vi "JKI Temelate.vi"() -> ()   [LabVIEW 2021]
uses:
  <userlib>/sushu/sushu.lvlib
panel:
  out "error out":errorcluster
  in  "error in (no error)":errorcluster
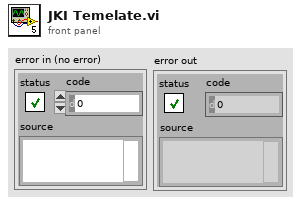
[diagram p1: front panel]
types:
  T1 = cluster{"Core":cluster{"Current VI Reference":refnum<vi>, "Close Panel on Exit?":bool}, "VI Name":string}
  T2 = enum32{"Invalid", "Standard", "Closed", "Hidden", "Minimized", "Maximized"}
  T3 = enum32{"invalid app kind", "Development System", "Run Time System", "Student Edition", "Embedded LabVIEW", "Evaluation", "Custom"}
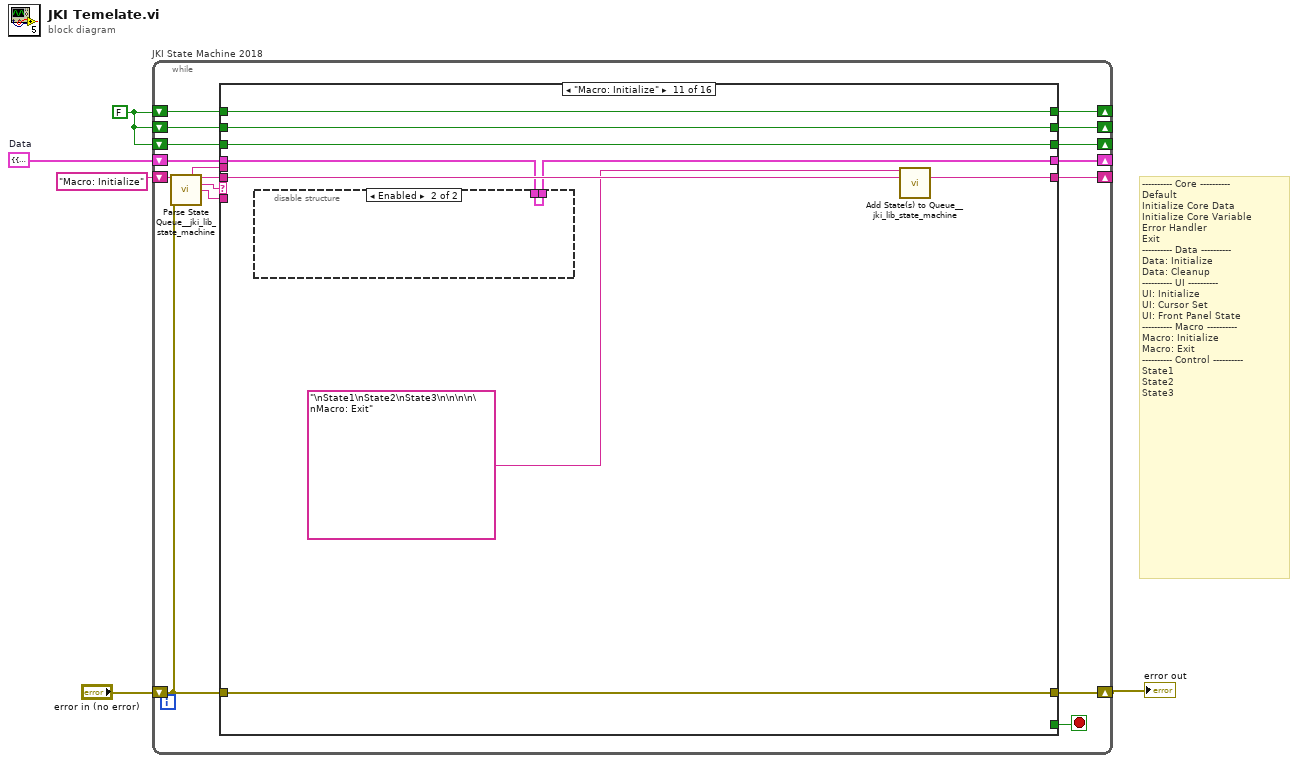
[diagram p0: block diagram]
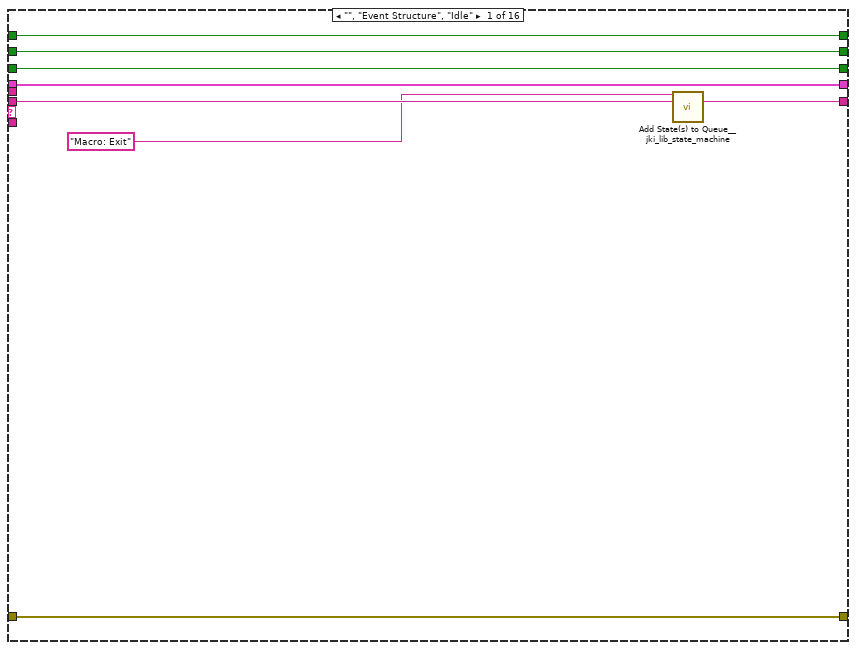
[diagram p2: hidden frame]
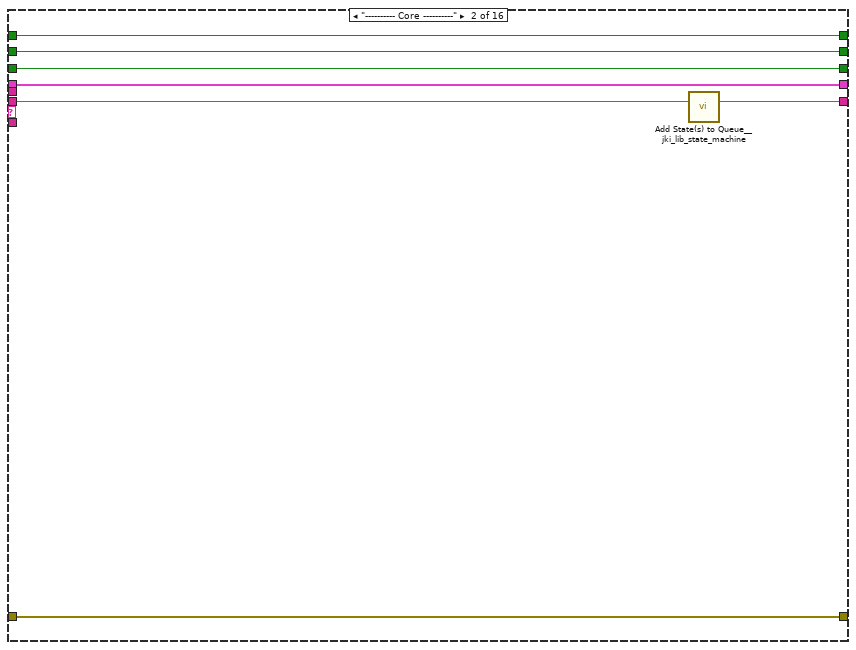
[diagram p3: hidden frame]
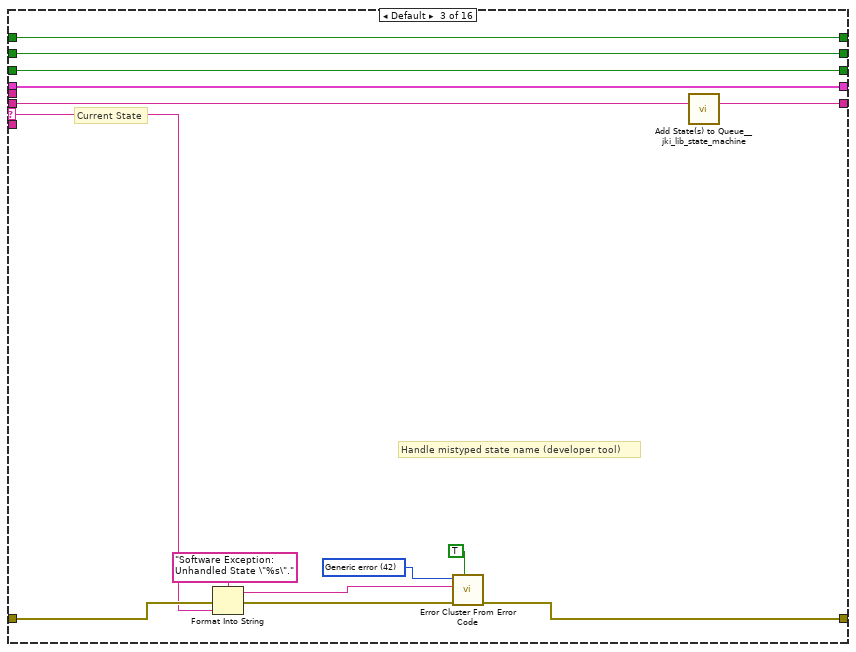
[diagram p4: hidden frame]
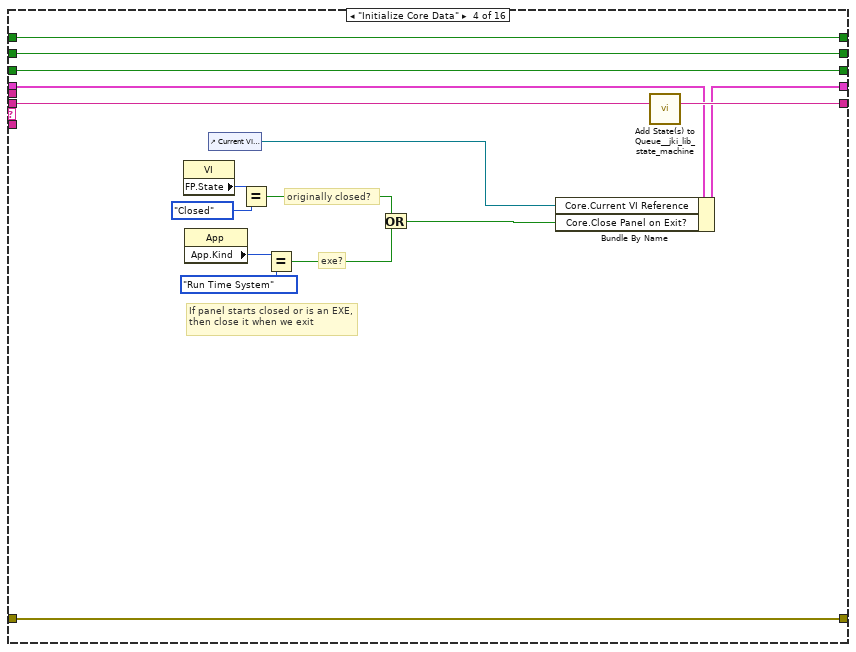
[diagram p5: hidden frame]
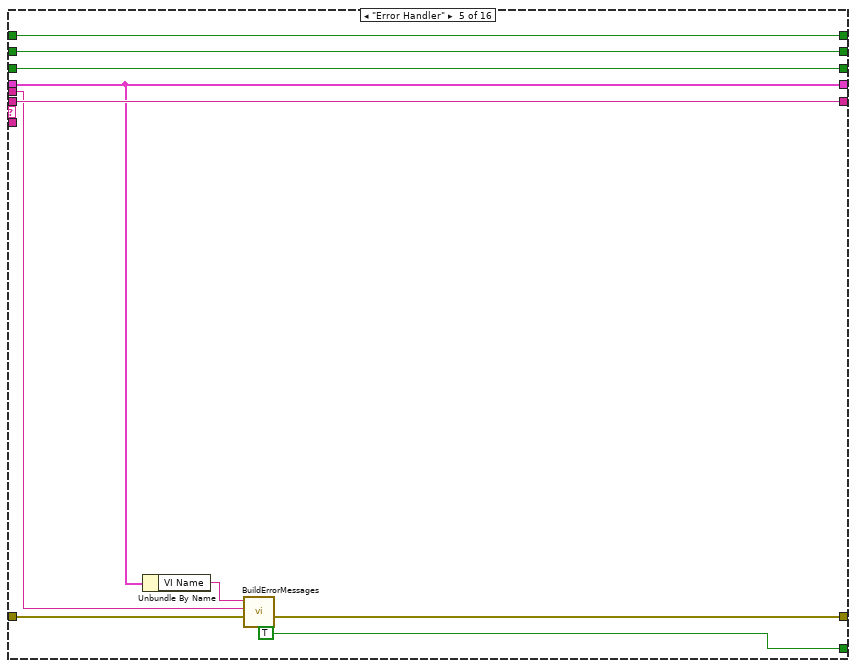
[diagram p6: hidden frame]
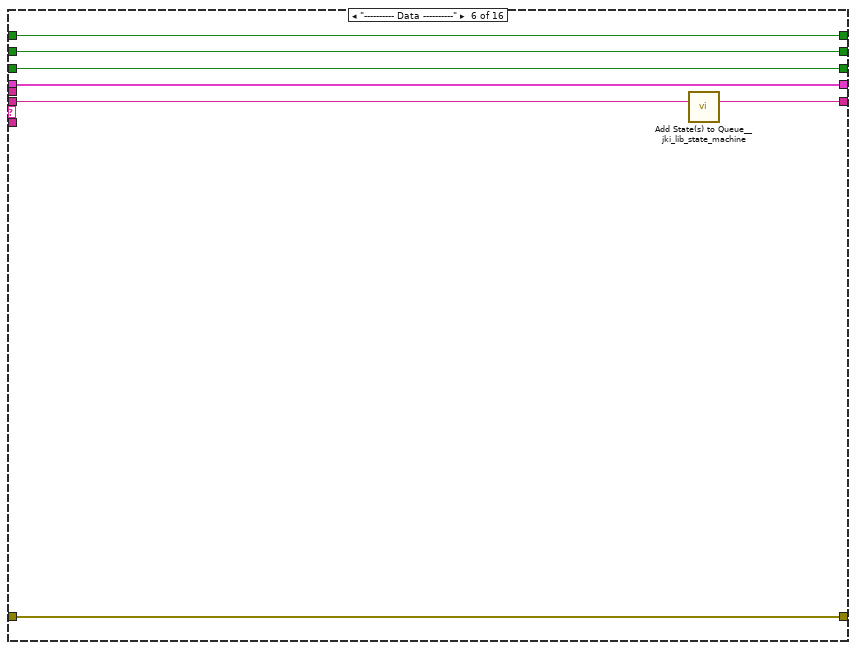
[diagram p7: hidden frame]
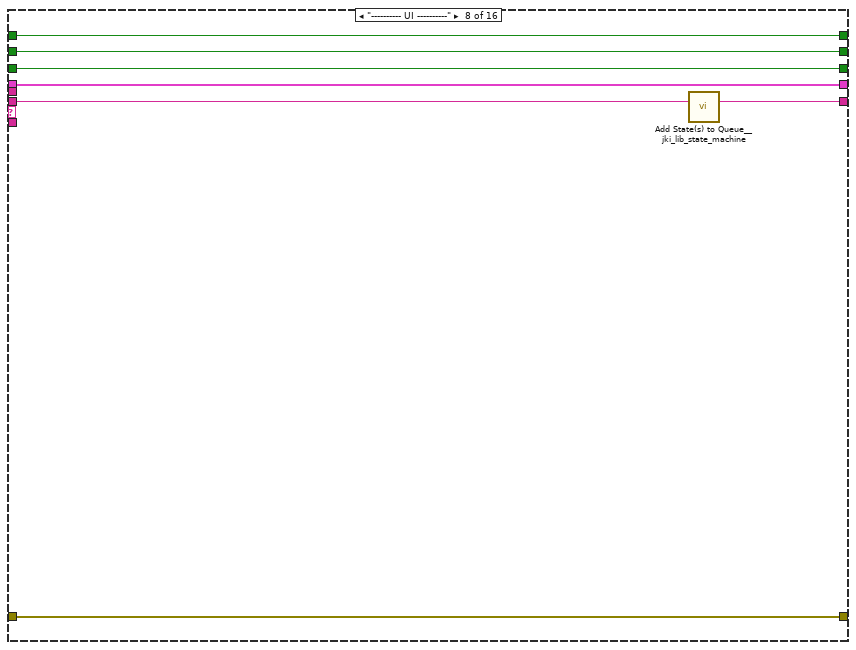
[diagram p9: hidden frame]
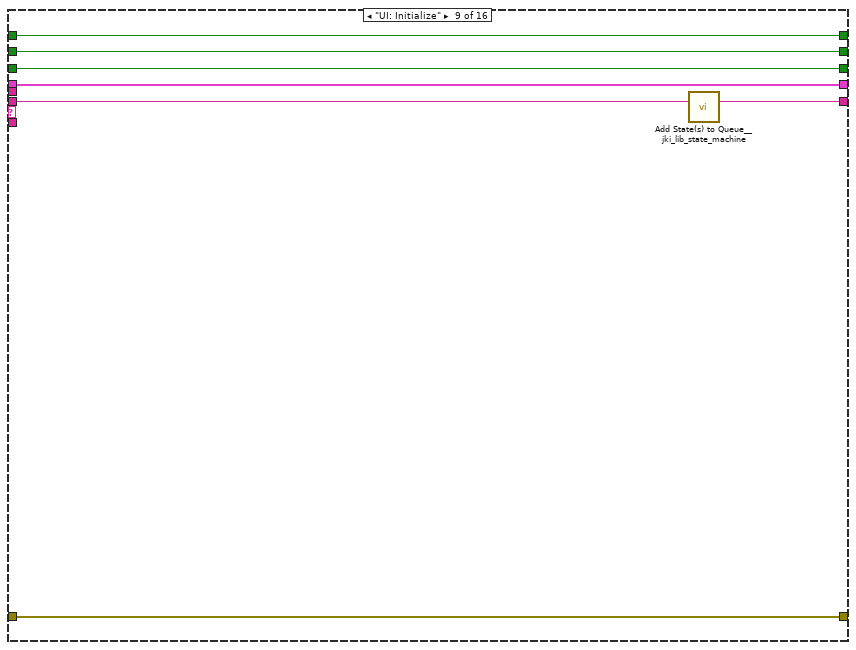
[diagram p10: hidden frame]
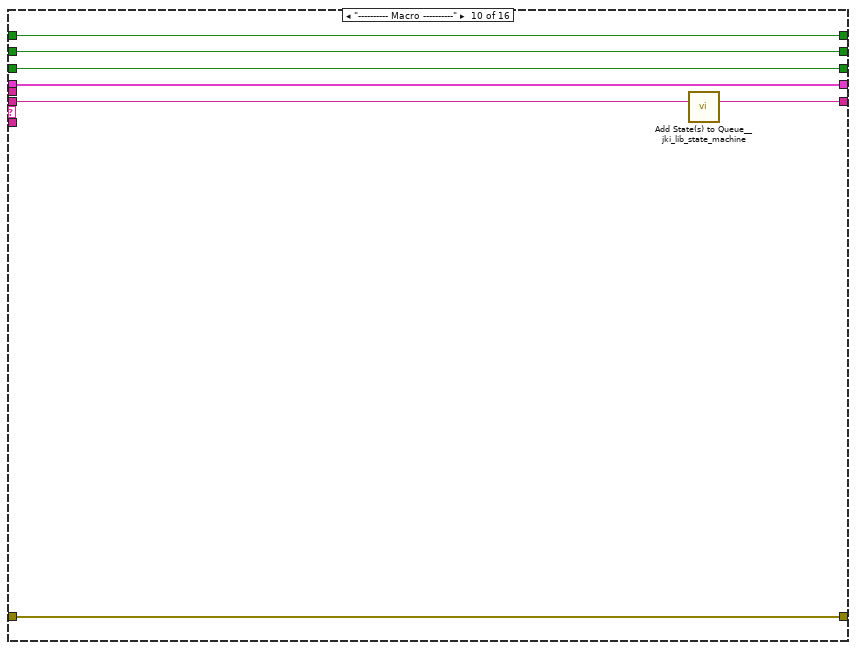
[diagram p11: hidden frame]
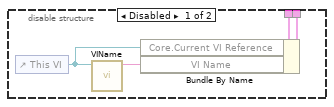
[diagram p12: hidden frame]
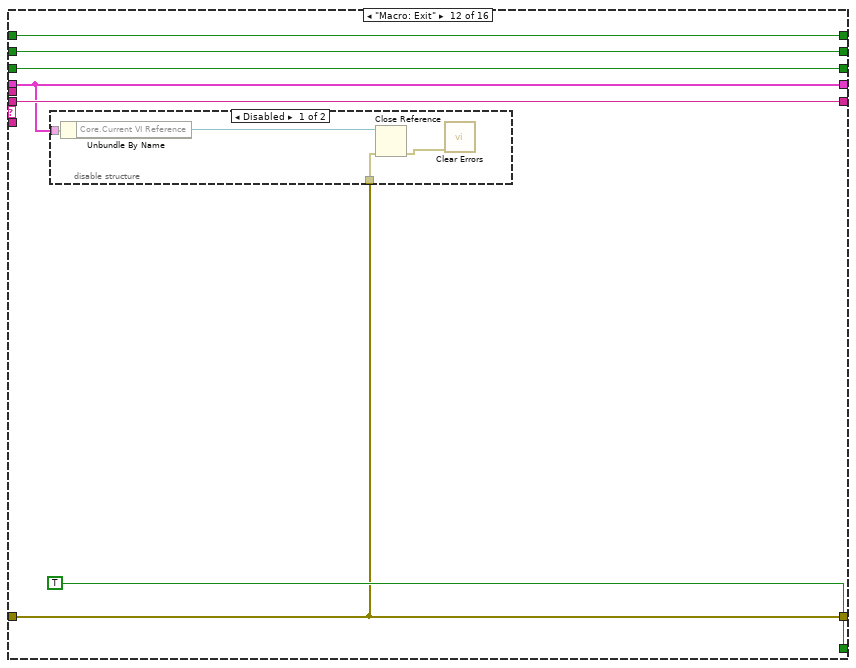
[diagram p13: hidden frame]
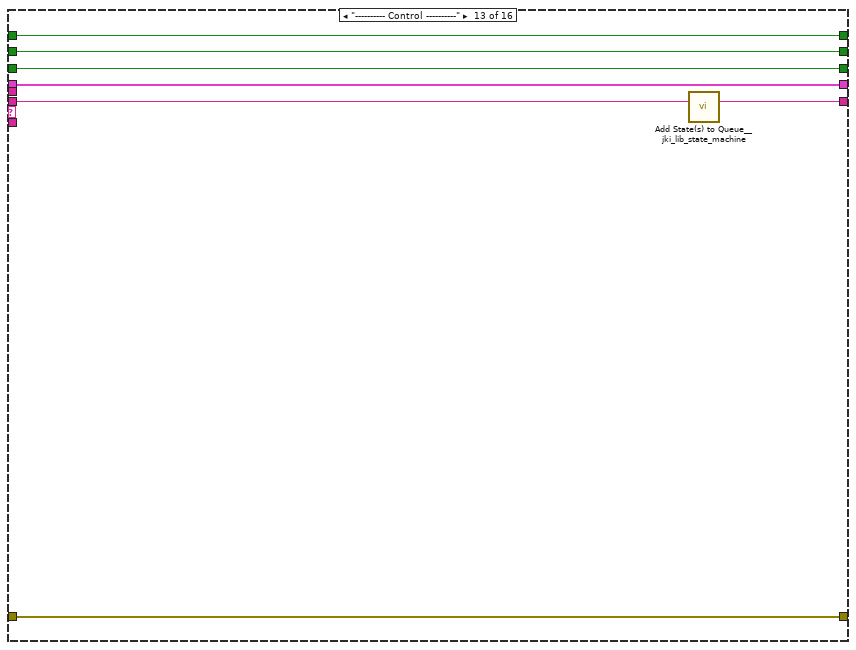
[diagram p15: hidden frame]
diagram:
  w1 = FALSE
  w2 = T1 {"Core"={"Current VI Reference"=refnum, "Close Panel on Exit?"=FALSE}, "VI Name"=""}  # Data
  # "---------- Core ----------\nDefault\nInitialize Core Data\nInitialize Core Variable\nError Handler\nExit\n---------- Data ----------\nData: Initialize\nData: Cleanup\n---------- UI ----------\nUI: Initialize\nUI: Cursor Set\nUI: Front Panel State\n---------- Macro ----------\nMacro: Initialize\nMacro: Exit\n---------- Control ----------\nState1\nState2\nState3"
  n1 = while "JKI State Machine 2018" {
    shift-right: [w16] -> _
    shift-left: w2 -> [w15]
    shift-right: [w19] -> w3
    shift-left: "error in (no error)" -> [w14]
    shift-right: [w18] -> _
    shift-left: "Macro: Initialize" -> [w20]
    shift-right: [w12] -> _
    shift-left: w1 -> [w13]
    shift-right: [w10] -> _
    shift-left: w1 -> [w6]
    shift-right: [w8] -> _
    shift-left: w1 -> [w9]
    stop <- w17 stop-if-true
    n2 = call <vilib>:"Parse State Queue__jki_lib_state_machine.vi"("State Queue"=w20, "Error In (no error)"=w14) -> ("Previous State"=w7:string, "Remaining States"=w22:string, "Current State"=w11:string, "Arguments"=w21:string)  [unwired: 10 in]
    n3 = case shown="\"Macro: Initialize\"" w11 {
      selector: w11 -> [_ _ w41 _ _ _ _ _ _ _ _ _ _ _ _ _]
      tunnel: w22 -> [w30 w37 w45 w67 w76 w84 w87 w97 w104 w111 w120 w130 w143 w149 w154 w160]
      tunnel: w21 -> [_ _ _ _ _ _ _ _ _ _ _ _ _ _ _ _]
      tunnel: w15 -> [w27 w34 w43 w60 w73 w81 w88 w94 w102 w108 w118 w128 w140 w148 w153 w159]
      tunnel: [w28 w35 w47 w64 w69 w82 w90 w95 w101 w109 w113 w127 w141 w145 w155 w161] -> w19
      tunnel: w14 -> [w28 w35 w46 w64 w70 w82 w90 w95 w101 w109 w113 w127 w141 w145 w155 w161]
      tunnel: [w29 w36 w44 w66 w76 w83 w87 w96 w103 w110 w119 w130 w142 w149 w154 w160] -> w18
      tunnel: [_ _ _ _ TRUE _ _ _ _ _ _ TRUE _ _ _ _] -> w17
      tunnel: [w27 w34 w43 w65 w73 w81 w88 w94 w102 w108 w115 w128 w140 w148 w153 w159] -> w16
      tunnel: w13 -> [w26 w33 w40 w54 w75 w80 w89 w93 w100 w107 w117 w132 w139 w147 w152 w158]
      tunnel: [w26 w33 w40 w54 w75 w80 w89 w93 w100 w107 w117 w132 w139 w147 w152 w158] -> w12
      tunnel: w6 -> [w25 w32 w39 w53 w74 w79 w86 w92 w99 w106 w114 w131 w138 w146 w151 w157]
      tunnel: [w25 w32 w39 w53 w74 w79 w86 w92 w99 w106 w114 w131 w138 w146 w151 w157] -> w10
      tunnel: w7 -> [_ _ _ _ w71 _ _ _ _ _ _ _ _ _ _ _]
      tunnel: w9 -> [w23 w31 w38 w52 w68 w78 w85 w91 w98 w105 w112 w126 w137 w144 w150 w156]
      tunnel: [w23 w31 w38 w52 w68 w78 w85 w91 w98 w105 w112 w126 w137 w144 w150 w156] -> w8
      frame "", "Event Structure", "Idle" {
        n4 = call <vilib>:"Add State(s) to Queue__jki_lib_state_machine.vi"("State(s) in Front (\"\")"="Macro: Exit" ("State(s) in Front (\"\")"), "State(s) in (\"\")"=w30) -> ("States Out"=w29:string)  [unwired: 13 in]
      }
      frame "---------- Core ----------" {
        n5 = call <vilib>:"Add State(s) to Queue__jki_lib_state_machine.vi"("State(s) in (\"\")"=w37) -> ("States Out"=w36:string)  [unwired: 14 in]
      }
      frame Default {
        w50 = 42 items=["No error", "Argument error", "Memory is full", "Out of zone", "End of file", "File already open", "Generic file I/O error", "File not found", "File permission error", "Disk is full", "Duplicate path", "Too many files open", "System feature not enabled", "Resource file not found", "Cannot add resource", "Resource not found", "Image not found", "Image memory error", "Pen does not exist", "Config type invalid", "Config token not found", "Config parse error", "Config memory error", "Bad external code format", "Bad external code offset", "External code not present", "Null window", "Destroy window error", "Null menu", "Print aborted", "Bad print record", "Print driver error", "Windows error during printing", "Memory error during printing", "Print dialog error", "Generic print error", "Invalid device refnum", "Device not found", "Device parameter error", "Device unit error", "Cannot open device", "Device call aborted", "Generic error", "Cancelled by user", "Object ID too low", "Object ID too high", "Object not in heap", "Unknown heap", "Unknown object (invalid DefProc)", "Unknown object (DefProc not in table)", "Message out of range", "Invalid (null) method", "Unknown message", "Manager call not supported", "Bad address", "Network operation in progress", "Network operation timed out", "Connection is busy", "Network attribute not supported", "Network error", "Address in use", "System out of memory", "Connection aborted", "Connection refused", "Not connected", "Already connected", "Connection closed", "Initialization error (interapplication manager)", "Bad occurrence", "Wait on unbound occurrence handler", "Occurrence queue overflow", "Datalog type conflict", "Unused", "Unrecognized type (interapplication manager)", "Memory corrupt", "Failed to make temporary DLL", "Old CIN version", "Drag socket not found", "Failed to load drop-object", "Failed to register OLE object", "Failed to release OLE object", "Format specifier type mismatch", "Unknown format specifier", "Too few format specifiers", "Too many format specifiers", "Scan failed", "Newer CIN version", "Error converting to variant", "Runtime menu error", "Password tampered", "Variant attribute not found", "Incompatible variant data type", "Event data is not available", "Event Store is not present", "Occurrence is not found", "Event Queue is not created", "Event info is not available", "Refnum passed is NULL", "Error retrieving Class GUID", "Error retrieving CoClass GUID", "Error retrieving TypeLib GUID.", "Bad built application magic bytes.", "Specific driver is different from the specific driver associated with the Logical Name.", "There is no session opened to the class driver.", "Max Error", "MAX - Error with config objects", "MAX - Error loading configuration", "MAX - Group not supported"]
        # "Current State"
        # "Handle mistyped state name (developer tool)"
        n6 = Format Into String(format string="Software Exception: Unhandled State \"%s\"." ("message"), error in=w46, w41) -> (resulting string=w49:string, error out=w48:errorcluster)  [unwired: 1 in]
        n7 = call <vilib>:"Error Cluster From Error Code.vi"("show call chain? (False)"=TRUE, "error in (no error)"=w48, "error message (\"\")"=w49, "error code (0)"=w50) -> ("error out"=w47:errorcluster)  [unwired: 5 in]
        n8 = call <vilib>:"Add State(s) to Queue__jki_lib_state_machine.vi"("State(s) in (\"\")"=w45) -> ("States Out"=w44:string)  [unwired: 14 in]
      }
      frame "Initialize Core Data" {
        # "originally closed?"
        # "exe?"
        # "If panel starts closed or is an EXE, then close it when we exit"
        n9 = property class="VI"() -> ("FP.State"=w57:T2)  [unwired: 2 in, 2 out]
        n10 = property class="App"() -> ("App.Kind"=w63:T3)  [unwired: 2 in, 2 out]
        n11 = control-ref of="Current VI Reference"() -> (w58:refnum<vi>)
        n12 = Equal?(x=w57, y=T2."Closed" ("Front Panel Window:State")) -> (x = y?=w55:bool)
        n13 = Equal?(x=w63, y=T3."Run Time System" ("Application:Kind")) -> (x = y?=w61:bool)
        n14 = Or(x=w55, y=w61) -> (x .or. y?=w59:bool)
        n15 = Bundle By Name(cluster=w60, "Core.Current VI Reference"=w58, "Core.Close Panel on Exit?"=w59) -> (w65:T1)
        n16 = call <vilib>:"Add State(s) to Queue__jki_lib_state_machine.vi"("State(s) in (\"\")"=w67) -> ("States Out"=w66:string)  [unwired: 14 in]
      }
      frame "Error Handler" {
        n17 = Unbundle By Name(w73) -> ("VI Name"=w72:string)
        n18 = call <userlib>:"BuildErrorMessages.vi"("error in"=w70, "ErrorCase"=w71, "VI Name"=w72) -> ("error out (no error)"=w69:errorcluster)  [unwired: 6 in, 2 out]
      }
      frame "---------- Data ----------" {
        n19 = call <vilib>:"Add State(s) to Queue__jki_lib_state_machine.vi"("State(s) in (\"\")"=w84) -> ("States Out"=w83:string)  [unwired: 14 in]
      }
      frame "Data: Initialize" {
      }
      frame "---------- UI ----------" {
        n20 = call <vilib>:"Add State(s) to Queue__jki_lib_state_machine.vi"("State(s) in (\"\")"=w97) -> ("States Out"=w96:string)  [unwired: 14 in]
      }
      frame "UI: Initialize" {
        n21 = call <vilib>:"Add State(s) to Queue__jki_lib_state_machine.vi"("State(s) in (\"\")"=w104) -> ("States Out"=w103:string)  [unwired: 14 in]
      }
      frame "---------- Macro ----------" {
        n22 = call <vilib>:"Add State(s) to Queue__jki_lib_state_machine.vi"("State(s) in (\"\")"=w111) -> ("States Out"=w110:string)  [unwired: 14 in]
      }
      frame "Macro: Initialize" {
        n23 = disable-structure shown="Enabled" {
          disable-tunnel: w118 -> [w124 w125]
          disable-tunnel: [w123 w125] -> w115
          frame Disabled {
            n24 = control-ref of="This VI"() -> (w121:refnum<vi>)
            n25 = call <userlib>:"VIName.vi"("reference"=w121) -> ("VI Name"=w122:string)  [unwired: 9 in, 1 out]
            n26 = Bundle By Name(cluster=w124, "Core.Current VI Reference"=w121, "VI Name"=w122) -> (w123:T1)
          }
          frame Enabled {
          }
        }
        n27 = call <vilib>:"Add State(s) to Queue__jki_lib_state_machine.vi"("State(s) in Front (\"\")"="\nState1\nState2\nState3\n\n\n\n\nMacro: Exit", "State(s) in (\"\")"=w120) -> ("States Out"=w119:string)  [unwired: 13 in]
      }
      frame "Macro: Exit" {
        n28 = disable-structure shown="Disabled" {
          disable-tunnel: w128 -> [w136 _]
          disable-tunnel: w127 -> [w134 _]
          frame Disabled {
            n29 = Unbundle By Name(w136) -> ("Core.Current VI Reference"=w135:refnum<vi>)
            n30 = Close Reference(reference=w135, error in (no error)=w134) -> (error out=w133:errorcluster)
            n31 = call <vilib>:"Clear Errors.vi"("error in (no error)"=w133) -> ()  [unwired: 5 in, 2 out]
          }
          frame Enabled {
          }
        }
      }
      frame "---------- Control ----------" {
        n32 = call <vilib>:"Add State(s) to Queue__jki_lib_state_machine.vi"("State(s) in (\"\")"=w143) -> ("States Out"=w142:string)  [unwired: 14 in]
      }
      frame "State1" {
      }
      frame "State2" {
      }
      frame "State3" {
      }
    }
  }
  "error out" <- w3
